vi "Sort Sync Mask with Schedules.vi"(8 "error in (no error)":errorcluster, 11 "Tamer in":refnum<class "Tamer.lvclass">) -> (0 "error out":errorcluster, 3 "Tamer out":refnum<class "Tamer.lvclass">)   [LabVIEW 2020, in "TALOS.lvlib" / "Tamer.lvlib" / "Tamer.lvclass"]
uses:
  Tamer.lvclass
  Tamer.lvclass/Tamer.ctl
  Ancestor/Ancestor/Ancestor.lvclass/Ancestor.ctl
  1905bdb5-c98e-4c40-a05c-e821c862ae70.vi
  FGV/Error Memory/Get Error Description.vi
  Support VIs/Get PC name.vi
  Ancestor/Ancestor/Read ID.vi
  Support VIs/Get Class Name.vi
  <vilib>/Utility/error.llb/Clear Errors.vi
  FGV/Error Memory/Error Memory Core.vi
  <vilib>/AdvancedString/Delimited String to 1D String Array.vi
  Support VIs/Circus Root Path.vi
  FGV/Error Memory/Error Crt Lvl checker.vi
  FGV/Error Memory/Error Memory Core.vi/40c8088d-b597-4017-91af-faa98e00292e.vi
  FGV/Error Memory/Error Memory Core.vi/d4a3ab98-063c-4e44-b43d-fbdcfe6c2be2.vi
  Support VIs/Global Memory.vi
  <vilib>/Utility/LVClass/Get LV Class Name.vi
  Support VIs/Is in Packed Library.vi
  Support VIs/TALOS Root path.vi
  Support VIs/Read CSV worksheet.vi
  Support VIs/Global Constants.vi
  <vilib>/Utility/error.llb/General Error Handler.vi
  <vilib>/Comparison/Less/Less Functor/Less Functor.lvclass
  Ancestor/Ancestor/Ancestor.lvclass
  <vilib>/Comparison/Equal/Equal Functor/Equal Functor.lvclass
  Run Utilities/Schedule/Schedule.lvclass
  TALOS.lvlib
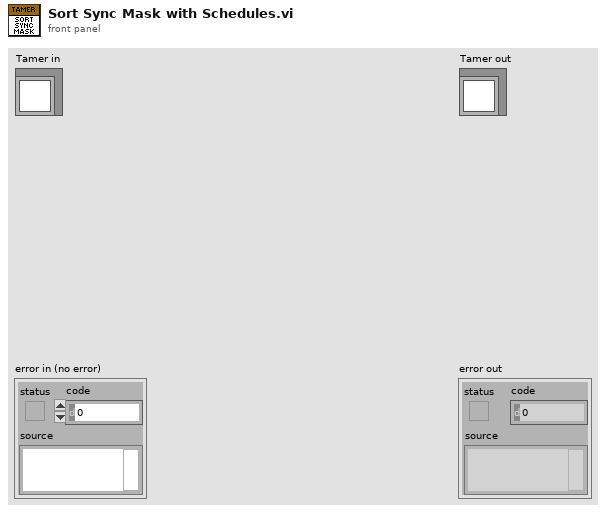
[diagram p1: front panel]
types:
  T1 = typedef "TALOS.lvlib/Run Utilities.lvlib/Synchronize FPGA Cluster.ctl" = cluster{"Status":bool, "FPGA Name":string}
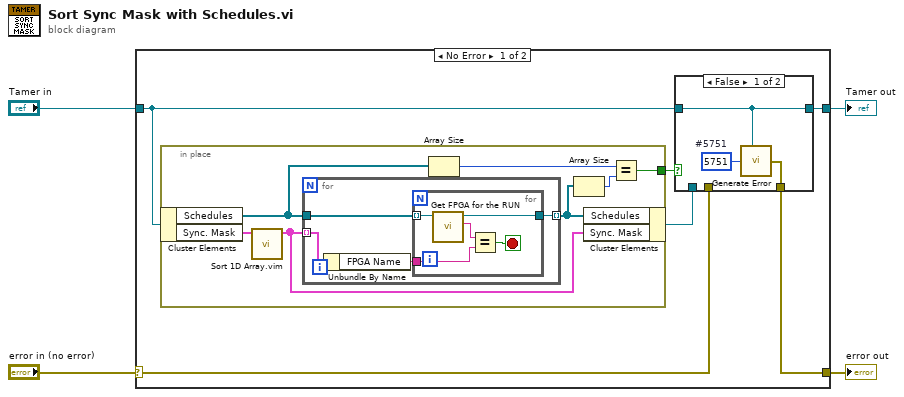
[diagram p0: block diagram]
diagram:
  n1 = case shown="No Error" "error in (no error)" {
    selector: "error in (no error)" -> [w5 w33]
    tunnel: [w6 w33] -> w3
    tunnel: [w8 w32] -> w1
    tunnel: "Tamer in" -> [w7 w32]
    frame No Error {
      n2 = in-place {
        in-place-border: [w17] -> w10
        n3 = in-place-cluster #1(w7) -> ("Schedules"=w21:refnum<class "Schedule.lvclass">[], "Sync. Mask"=w16:T1[])
        n4 = call "Sort 1D Array.vim"("unsorted array"=w16) -> ("sorted array"=w22:T1[])  [unwired: 10 in]
        n5 = for {
          tunnel: w21 -> [w25]
          tunnel: w22 -> [w26] mode=indexing
          tunnel: [w23] -> w18 mode=indexing
          n6 = Unbundle By Name(w26) -> ("FPGA Name"=w24:string)
          n7 = for {
            tunnel: w25 -> [w31] mode=indexing
            tunnel: w24 -> [w29]
            tunnel: [w27] -> w23
            stop <- w28 stop-if-true
            n8 = call-dynamic "Get FPGA for the RUN.vi"("Schedule in"=w31) -> ("FPGA Name"=w30:string, "Schedule out"=w27:refnum<class "Schedule.lvclass">)  [unwired: 8 in, 1 out]
            n9 = Equal?(x=w30, y=w29) -> (x = y?=w28:bool)
          }
        }
        n10 = Array Size(array=w21) -> (size(s)=w20:i32)
        n11 = Array Size(array=w18) -> (size(s)=w19:i32)
        n12 = in-place-cluster #1("Schedules"=w18, "Sync. Mask"=w22) -> (w9:refnum<class "Tamer.lvclass">)
        n13 = Equal?(x=w20, y=w19) -> (x = y?=w17:bool)
      }
      n14 = case shown="False" w10 {
        tunnel: w9 -> [_ w15]
        tunnel: [w13 w15] -> w8
        tunnel: w7 -> [w13 _]
        tunnel: [w12 w14] -> w6
        tunnel: w5 -> [_ w14]
        frame False {
          w11 = 5751  # #5751
          n15 = call "Generate Error.vi"("Class"=w13, "Error Code"=w11) -> ("error out"=w12:errorcluster)  [unwired: 5 in]
        }
        frame True {
        }
      }
    }
    frame Error {
    }
  }
  "error out" <- w3
  "Tamer out" <- w1
